vi "System Monitoring Loop.vi"(8 "error in (no error)":errorcluster) -> ()   [LabVIEW 2014]
uses:
  RT Stop.vi
  RT Tags.vi
  <resource>/objmgr/nisysapi.rc
  <vilib>/NI_Real-Time Target Support.lvlib
  <vilib>/nisyscfg/nisyscfg.lvlib
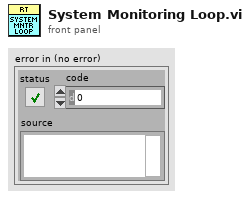
[diagram p1: front panel]
types:
  T1 = typedef "NI_Real-Time Target Support.lvlib/RT CPU Load.ctl" = cluster{"Total (%)":dbl, "Time Critical (%)":dbl, "Timed Structures (%)":dbl, "High (%)":dbl, "Above Normal (%)":dbl, "Normal (%)":dbl, "Background (%)":dbl, "Idle (%)":dbl, "ISR (%)":dbl}
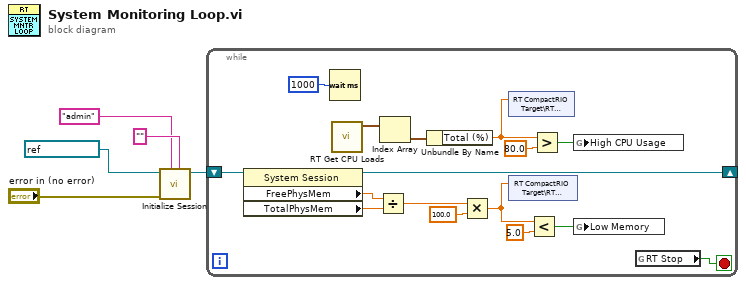
[diagram p0: block diagram]
diagram:
  n1 = call <vilib>:"Initialize Session.vi"("Password"="", "User Name"="admin", "error in (no error)"="error in (no error)", "Target (localhost)"=refnum<k21> "localhost") -> ("Session out"=w1:refnum<k21>)  [unwired: 6 in, 1 out]
  n2 = while {
    shift-right: [w19] -> _
    shift-left: w1 -> [w20]
    stop <- w21 stop-if-true
    n3 = property class="System Session"(reference=w20) -> (reference out=w19:refnum<k21>, "FreePhysMem"=w18:dbl, "TotalPhysMem"=w17:dbl)  [unwired: 1 in, 1 out]
    n4 = Wait (ms)(milliseconds to wait=u32 1000) -> ()  [unwired: 1 out]
    n5 = call <vilib>:"RT Get CPU Loads.vi"() -> ("CPU loads"=w13:T1[])  [unwired: 10 in, 1 out]
    n6 = Divide(x=w18, y=w17) -> (x/y=w16:dbl)
    n7 = Index Array(array=w13) -> (element=w14:T1)  [unwired: 1 in]
    n8 = Unbundle By Name(w14) -> ("Total (%)"=w11:dbl)
    n9 = Multiply(x=w16, y=100.0) -> (x*y=w9:dbl)
    n10 = shared-variable "RT CompactRIO Target\\RT Variables.lvlib\\CPU"(w11) -> ()  [unwired: 1 in, 1 out]
    n11 = shared-variable "RT CompactRIO Target\\RT Variables.lvlib\\RAM"(w9) -> ()  [unwired: 1 in, 1 out]
    n12 = Less?(x=w9, y=5.0) -> (x < y?=w7:bool)
    n13 = Greater?(x=w11, y=80.0) -> (0:w6:bool)
    n14 = global write "RT Tags.vi" "High CPU Usage"(w6) -> ()
    n15 = global write "RT Tags.vi" "Low Memory"(w7) -> ()
    n16 = global read "RT Stop.vi" "RT Stop"() -> (w21:bool)
  }
